vi "oscRLS.vi"(1 "u4":sgl, 2 "u3":sgl, 3 "u2":sgl, 4 "u1":sgl) -> (0 "f(u)":sgl)   [LabVIEW 2013]
panel:
  # "This VI is configured as Non-reentrant. \nOnly ONE copy of the Vi actually exists on the FPGA hardware."
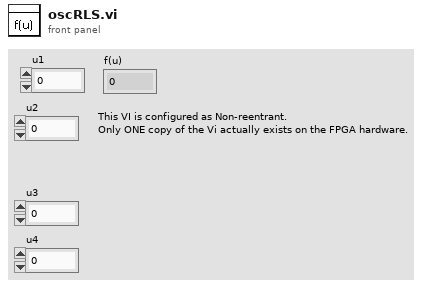
[diagram p1: front panel]
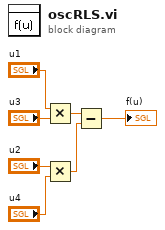
[diagram p0: block diagram]
diagram:
  n1 = Multiply(x="u1", y="u3") -> (x*y=w3:sgl)
  n2 = Multiply(x="u2", y="u4") -> (x*y=w2:sgl)
  n3 = Subtract(x=w3, y=w2) -> (x-y=→"f(u)":sgl)
